vi "get time ms 64.vi"(11 "dest":cluster{}) -> (2 "function return":u64, 3 "dest out":cluster{})   [LabVIEW 2019, in "apdm.lvlib"]
doc: "APDM_EXPORT uint64_t apdm_get_time_ms_64(struct timeval *dest);"
uses:
  apdm.lvlib
  Lee Lab/CP FES Walking 2018/Code/Working/LabVIEW/apdm.dll
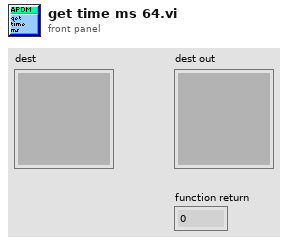
[diagram p1: front panel]
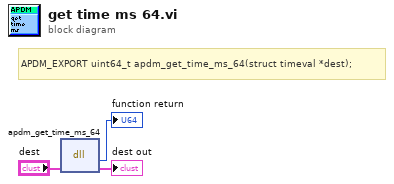
[diagram p0: block diagram]
diagram:
  # "APDM_EXPORT uint64_t apdm_get_time_ms_64(struct timeval *dest);"
  n1 = dll-call lib="C:/Users/jfalesi/Dropbox/Lee Lab/CP FES Walking 2018/Code/Working/LabVIEW/apdm.*" fn="apdm_get_time_ms_64"("dest"="dest") -> (→"function return":u64, "dest"=→"dest out":cluster{})  [unwired: 3 in, 2 out]
